vi "_Main_ByRuns_DAC2022_V1.0.1.vi"() -> ()   [LabVIEW 2017]
uses:
  <vilib>/Instr/_visa.llb/VISA Configure Serial Port (Instr).vi
panel:
  out "Field, kV/cm":dbl
  out "Current, mA":dbl
  out "Voltage, V":dbl
  in  "COM DAC":refnum<visa-resource-name>
  in  "WaveForm":i32(listbox)
  in  "Auto\nturn OFF":bool
  in  "Content":i32(listbox)
  out "LastTrigTimer, s":dbl
  in  "Graph every, cycle":dbl=10.0 min=1.0 max=100.0
  in  "SendPeriod, ms":dbl=100.0 min=10.0 max=10000.0
  out "RunsNeed":i32
  out "Time LOG":cluster{dbl[], dbl[]}(graph)
  out "TrigTimer, s":dbl
  out "Bytes at Port":u32
  out "RecTry":i32
  out "OutVoltage, V":dbl
  in  "Exposition, s":dbl=3.0
  out "Channel 2, V":dbl format="%#_5g"
  out "Channel 1, V":dbl format="%#_5g"
  in  "Stop Button":bool
  in  "Start Button":bool
  in  "Sample H, um":dbl=32.0
  out "VoltageArray, V":dbl[](array[numeric])
  out "Shutter Red":bool
  out "Shutter Green":bool
  in  "Frames In Run":u32=180
  out "Global Frame Done":u32
  out "Now is Run #":u32
  out "Frame In Run Done":u32
  in  "Step, kV/cm":dbl=1.0 min=0.01 max=1000.0
  in  "Amplitude, kV/cm":dbl=10.0 min=10.0 max=1500.0
  in  "LOG file":path
  in  "COM ADC":refnum<visa-resource-name>
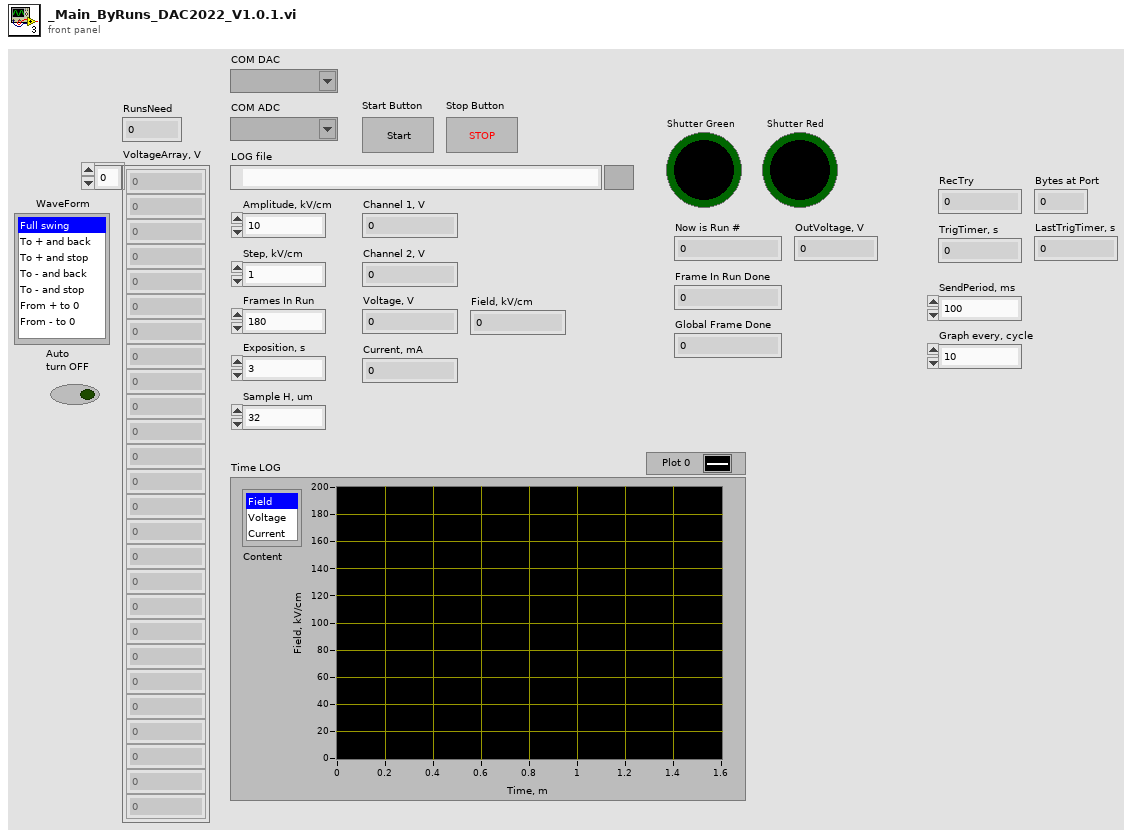
[diagram p1: front panel]
types:
  T1 = cluster{i32, i32, u32, "TrigState":bool, "TrigTimer, s":dbl, "CurrentError":bool}
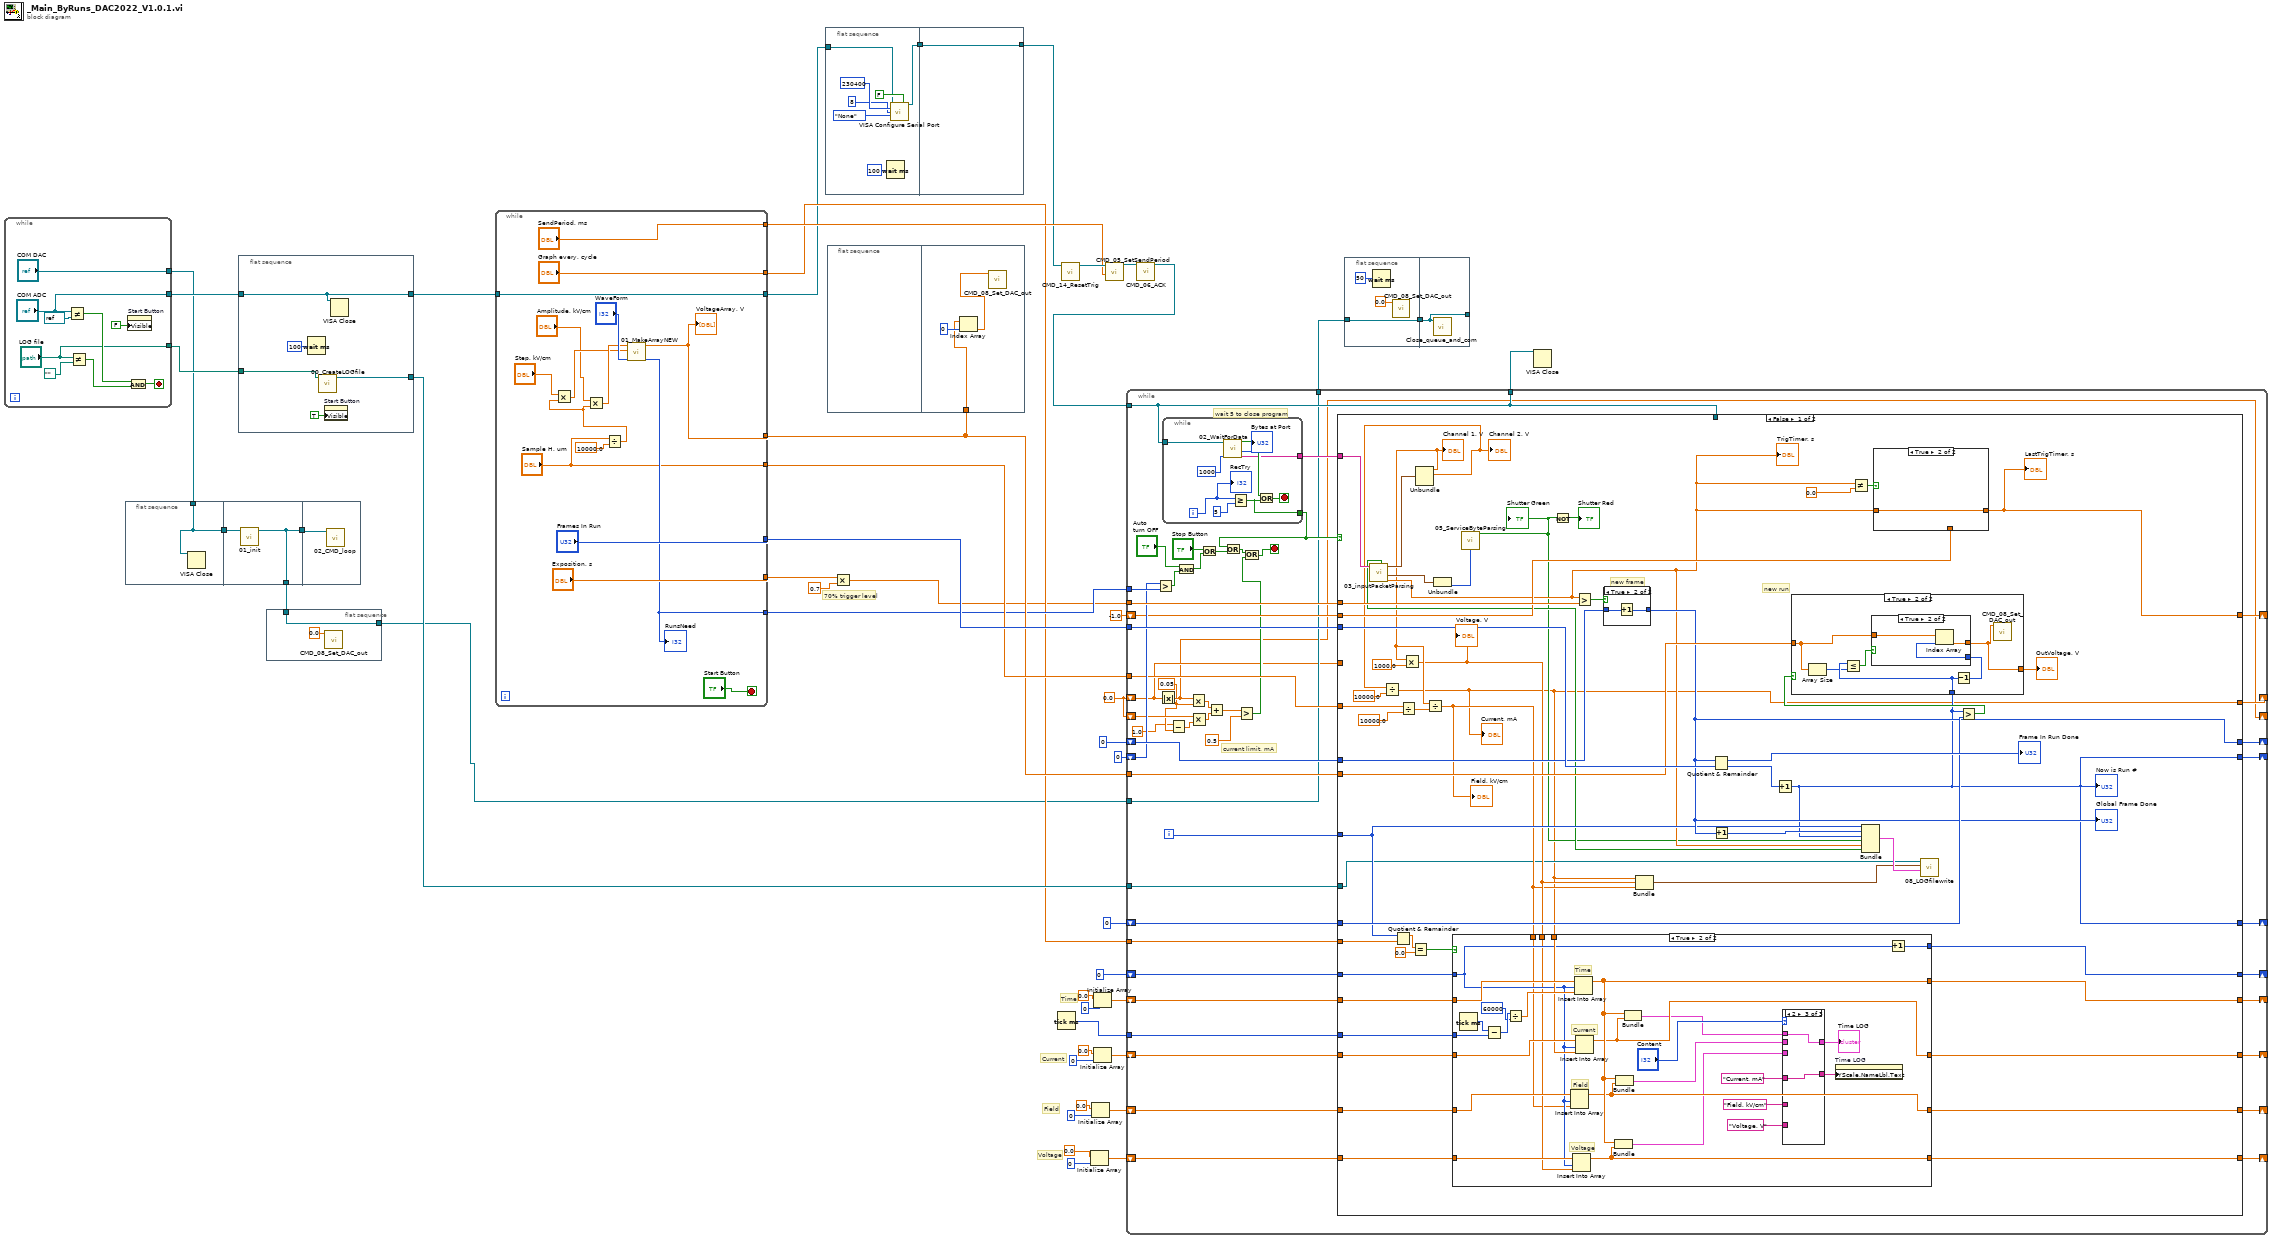
[diagram p0: block diagram]
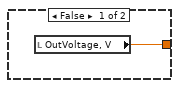
[diagram p6: hidden frame]
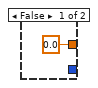
[diagram p7: hidden frame]
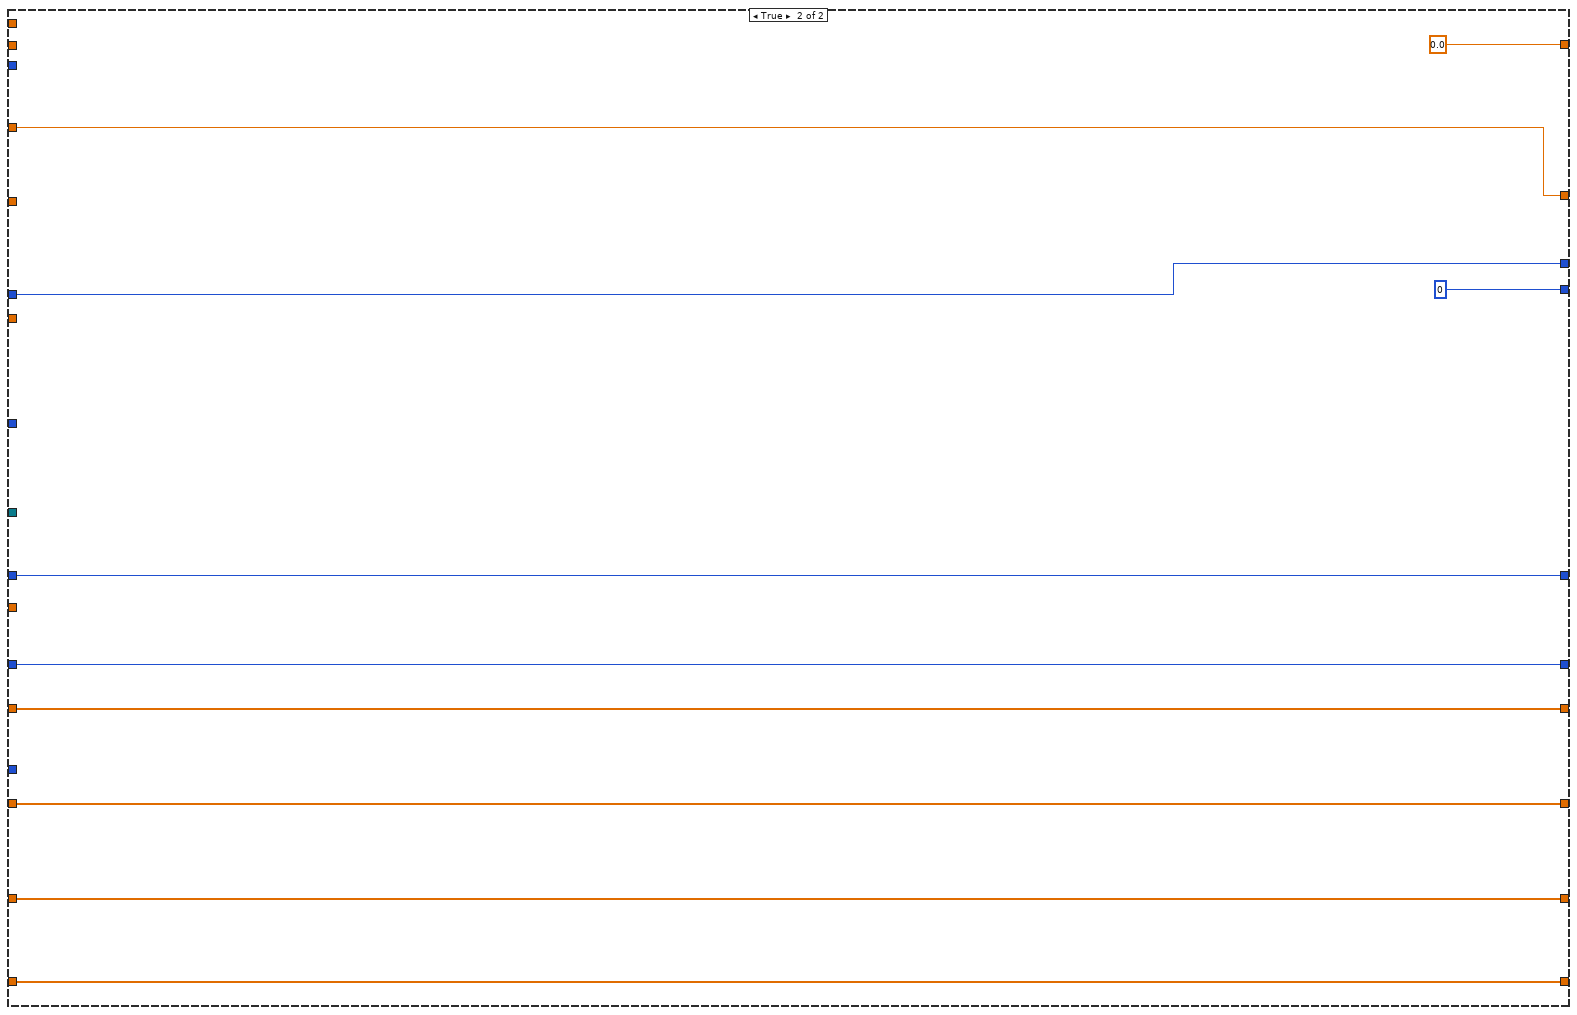
[diagram p9: hidden frame]
diagram:
  w1 = 0.0
  # "70% trigger level"
  # "Voltage"
  # "Field"
  # "Time"
  # "Current"
  n1 = while {
    tunnel: ["COM ADC"] -> w15
    tunnel: ["LOG file"] -> w14
    tunnel: ["COM DAC"] -> w6
    stop <- w53 stop-if-true
    n2 = Not Equal?(x="COM ADC", y=refnum<visa-resource-name> refnum ("COM port")) -> (x != y?=w50:bool)
    n3 = Not Equal?(x="LOG file", y=path "" ("LOG file")) -> (x != y?=w51:bool)
    n4 = property on="Start Button" class="Bool"("Visible"=FALSE) -> ()  [unwired: 2 in, 2 out]
    n5 = And(x=w50, y=w51) -> (x .and. y?=w53:bool)
  }
  n6 = flat-sequence {
    tunnel: [w56] -> w8
    tunnel: w6 -> [w56]
    tunnel: w8 -> [w58]
    tunnel: [w57] -> w5
    tunnel: [w57] -> w7
    tunnel: w7 -> [w59]
    frame #0 {
      n7 = VISA Close(VISA resource name=w56) -> ()  [unwired: 1 in, 1 out]
    }
    frame #1 {
      n8 = call "01_init.vi"("COM port"=w58) -> ("VISA resource name out"=w57:refnum<visa-resource-name>)  [unwired: 8 in, 2 out]
    }
    frame #2 {
      n9 = call "02_CMD_loop.vi"("VISA resource name"=w59) -> ()  [unwired: 11 in]
    }
  }
  n10 = flat-sequence {
    tunnel: [w64] -> w44
    tunnel: w15 -> [w60]
    tunnel: w14 -> [w61]
    tunnel: [w60] -> w13
    frame #0 {
      n11 = Wait (ms)(milliseconds to wait=u32 100) -> ()  [unwired: 1 out]
      n12 = call "00_CreateLOGfile.vi"("LOG file"=w61) -> ("refnum out"=w64:refnum<file>)  [unwired: 10 in]
      n13 = property on="Start Button" class="Bool"("Visible"=TRUE) -> ()  [unwired: 2 in, 2 out]
      n14 = VISA Close(VISA resource name=w60) -> ()  [unwired: 1 in, 1 out]
    }
  }
  n15 = flat-sequence {
    tunnel: w5 -> [w65]
    tunnel: [w65] -> w2
    frame #0 {
      n16 = call "CMD_08_Set_DAC_out.vi"("DAC voltage, V"=0.0) -> ()  [unwired: 11 in]
    }
  }
  n17 = while {
    tunnel: w13 -> [w76]
    tunnel: [w76] -> w11
    tunnel: [w75] -> w38
    tunnel: ["Sample H, um"] -> w45
    tunnel: ["Frames In Run"] -> w46
    tunnel: ["Exposition, s"] -> w24
    tunnel: [w74] -> w29
    tunnel: ["SendPeriod, ms"] -> w27
    tunnel: ["Graph every, cycle"] -> w26
    stop <- "Start Button" stop-if-true
    n18 = Divide(x="Sample H, um", y=10000.0) -> (x/y=w68:dbl)
    n19 = Multiply(x="Step, kV/cm", y=w68) -> (x*y=w70:dbl)
    n20 = Multiply(x="Amplitude, kV/cm", y=w68) -> (x*y=w71:dbl)
    n21 = call "01_MakeArrayNEW.vi"("Amp"=w71, "Step"=w70, "WaveForm"="WaveForm") -> ("Array"=w75:dbl[], "ArraySize"=w74:i32)  [unwired: 6 in]
    "VoltageArray, V" <- w75
    "RunsNeed" <- w74
  }
  n22 = flat-sequence {
    tunnel: w11 -> [w85]
    tunnel: [w84] -> w12
    tunnel: w12 -> [w90]
    tunnel: [w90] -> w10
    frame #0 {
      n23 = Wait (ms)(milliseconds to wait=u32 100) -> ()  [unwired: 1 out]
      n24 = call-poly "VISA Configure Serial Port"("VISA resource name"=w85, "Enable Termination\nChar (T)"=FALSE ("Enable Termination\nChar (T)"), "baud rate (9600)"=u32 230400, "data bits (8)"=u16 8, "parity (0:none)"=enum16{"None", "Odd", "Even", "Mark", "Space"}."None") -> ("VISA resource name out"=w84:refnum<visa-resource-name>)  [unwired: 9 in, 1 out]
    }
    frame #1 {
    }
  }
  n25 = flat-sequence {
    tunnel: w38 -> [w92]
    frame #0 {
    }
    frame #1 {
      n26 = Index Array(array=w92, index=0) -> (element=w91:dbl)
      n27 = call "CMD_08_Set_DAC_out.vi"("DAC voltage, V"=w91) -> ()  [unwired: 11 in]
    }
  }
  n28 = Multiply(x=w24, y=0.7) -> (x*y=w25:dbl)
  n29 = Tick Count (ms)() -> (millisecond timer value=w33:u32)
  n30 = call "CMD_14_ResetTrig.vi"("VISA resource name"=w10) -> ("VISA resource name out"=w41:refnum<visa-resource-name>)  [unwired: 10 in]
  n31 = Initialize Array(0.0 ("element"), 0 ("dimension size")) -> (w16:dbl[])
  n32 = Initialize Array(0.0 ("element"), 0 ("dimension size")) -> (w17:dbl[])
  n33 = Initialize Array(0.0 ("element"), 0 ("dimension size")) -> (w30:dbl[])
  n34 = Initialize Array(0.0 ("element"), 0 ("dimension size")) -> (w34:dbl[])
  n35 = call "CMD_05_SetSendPeriod.vi"("Period, ms"=w27, "VISA resource name"=w41) -> ("VISA resource name out"=w40:refnum<visa-resource-name>)  [unwired: 9 in]
  n36 = call "CMD_06_ACK.vi"("VISA resource name"=w40) -> ("VISA resource name out"=w39:refnum<visa-resource-name>)  [unwired: 10 in]
  n37 = while {
    tunnel: w39 -> [w110]
    tunnel: w38 -> [w133]
    tunnel: w46 -> [w139]
    tunnel: w25 -> [w141]
    tunnel: w45 -> [w111]
    tunnel: w44 -> [w140]
    shift-right: [w136] -> _
    shift-left: 0 -> [w138]
    shift-right: [w135] -> _
    shift-left: u32 0 -> [w134]
    shift-right: [w131] -> _
    shift-left: 0 -> [w132]
    tunnel: w33 -> [w129]
    shift-right: [w127] -> _
    shift-left: w34 -> [w130]
    shift-right: [w126] -> _
    shift-left: w30 -> [w128]
    tunnel: w29 -> [w122]
    shift-right: [w124] -> _
    shift-left: u32 0 -> [w121]
    tunnel: w26 -> [w118]
    shift-right: [w117] -> _
    shift-left: -1.0 ("TrigTimer, s") -> [w116]
    shift-right: [w113] -> _
    shift-left: w17 -> [w115]
    shift-right: [w112] -> _
    shift-left: w16 -> [w114]
    tunnel: [w109] -> w3
    tunnel: [w110] -> w9
    tunnel: w2 -> [w109]
    shift-right: [w108] -> _
    shift-left: w1 -> [w103]
    shift-right: [w102] -> _
    shift-left: w1 -> [w101]
    i -> [w137]
    stop <- w106 stop-if-true
    w99 = 0.05
    # "current limit, mA"
    # "wait 5 to close program"
    n38 = Greater?(x=w121, y=w122) -> (0:w119:bool)
    n39 = Absolute Value(x=w103) -> (abs(x)=w102:dbl)
    n40 = while {
      tunnel: w110 -> [w262]
      tunnel: [w265] -> w143
      tunnel: [w266] -> w142
      i -> [w264]
      stop <- w268 stop-if-true
      n41 = call "02_WaitForData.vi"("WaitTimeoutMS"=u32 1000, "VISA"=w262) -> ("Buffer"=w266:string, "Bytes at Port"=→"Bytes at Port":u32, "Data Recived"=w267:bool)  [unwired: 7 in]
      n42 = Greater Or Equal?(x=w264, y=5) -> (x >= y?=w265:bool)
      n43 = Or(x=w267, y=w265) -> (x .or. y?=w268:bool)
      "RecTry" <- w264
    }
    n44 = Subtract(x=1.0, y=w99) -> (x-y=w100:dbl)
    n45 = And(x="Auto\nturn OFF", y=w119) -> (x .and. y?=w120:bool)
    n46 = Multiply(x=w102, y=w99) -> (x*y=w96:dbl)
    n47 = Multiply(x=w101, y=w100) -> (x*y=w97:dbl)
    n48 = Or(x="Stop Button", y=w120) -> (x .or. y?=w125:bool)
    n49 = Add(x=w96, y=w97) -> (x+y=w95:dbl)
    n50 = Or(x=w143, y=w125) -> (x .or. y?=w105:bool)
    n51 = Greater?(x=w95, y=0.5) -> (0:w104:bool)
    n52 = Or(x=w105, y=w104) -> (x .or. y?=w106:bool)
    n53 = case shown="False" w143 {
      tunnel: w142 -> [w197 _]
      tunnel: w141 -> [w193 _]
      tunnel: w140 -> [w145 _]
      tunnel: w139 -> [w194 _]
      tunnel: w138 -> [w191 w261]
      tunnel: w137 -> [w178 _]
      tunnel: [w183 w261] -> w136
      tunnel: [w169 w260] -> w135
      tunnel: w134 -> [w186 w260]
      tunnel: w133 -> [w187 _]
      tunnel: w110 -> [_ _]
      tunnel: w132 -> [w176 w259]
      tunnel: [w175 w259] -> w131
      tunnel: w130 -> [w174 w258]
      tunnel: w129 -> [w173 _]
      tunnel: w128 -> [w172 w257]
      tunnel: [w171 w258] -> w127
      tunnel: [w170 w257] -> w126
      tunnel: [w169 u32 0] -> w124
      tunnel: w118 -> [w168 _]
      tunnel: [w165 0.0 ("TrigTimer, s")] -> w117
      tunnel: w116 -> [w164 _]
      tunnel: w115 -> [w160 w254]
      tunnel: w114 -> [w159 w253]
      tunnel: [w158 w254] -> w113
      tunnel: [w157 w253] -> w112
      tunnel: w111 -> [w151 _]
      tunnel: [w144 w252] -> w108
      tunnel: w103 -> [_ w252]
      frame False {
        # "new run"
        # "new frame"
        n54 = call "03_inputPacketParsing.vi"("string"=w197) -> ("TrigTimer, s"=w163:dbl, "Service state"=w182:cluster{u8, u8}, "Voltage"=w195:cluster{dbl, dbl, dbl, dbl}, "CurrentError"=w162:bool)  [unwired: 6 in, 1 out]
        "TrigTimer, s" <- w163
        n55 = Quotient & Remainder(x=w178, y=w168) -> (x-y*floor(x/y)=w180:dbl)  [unwired: 1 out]
        n56 = Divide(x=w151, y=10000.0) -> (x/y=w152:dbl)
        n57 = Equal?(x=w180, y=0.0) -> (x = y?=w177:bool)
        n58 = Unbundle(w195) -> (w153:dbl, w155:dbl)  [unwired: 2 out]
        "Channel 1, V" <- w153
        "Channel 2, V" <- w155
        n59 = Divide(x=w155, y=10000.0) -> (x/y=w144:dbl)
        "Current, mA" <- w144
        n60 = Multiply(x=w153, y=1000.0) -> (x*y=w148:dbl)
        "Voltage, V" <- w148
        n61 = Divide(x=w153, y=w152) -> (x/y=w147:dbl)
        "Field, kV/cm" <- w147
        n62 = Unbundle(w182) -> (w181:u8)  [unwired: 1 out]
        n63 = case shown="True" w177 {
          tunnel: w176 -> [w204 w220]
          tunnel: [w204 w227] -> w175
          tunnel: w174 -> [w202 w225]
          tunnel: w173 -> [_ w230]
          tunnel: w172 -> [w203 w224]
          tunnel: [w203 w216] -> w170
          tunnel: [w202 w219] -> w171
          tunnel: w144 -> [_ w223]
          tunnel: w160 -> [w201 w222]
          tunnel: w159 -> [w200 w221]
          tunnel: [w201 w217] -> w158
          tunnel: [w200 w218] -> w157
          tunnel: w148 -> [_ w206]
          tunnel: w147 -> [_ w205]
          frame False {
          }
          frame True {
            # "Time"
            # "Voltage"
            # "Field"
            # "Current"
            n64 = Tick Count (ms)() -> (millisecond timer value=w231:u32)
            n65 = Subtract(x=w231, y=w230) -> (x-y=w229:u32)
            n66 = Divide(x=w229, y=u32 60000) -> (x/y=w226:dbl)
            n67 = Insert Into Array(array=w222, index=w220, new element=w205) -> (w217:dbl[])
            n68 = Insert Into Array(array=w221, index=w220, new element=w206) -> (w218:dbl[])
            n69 = Insert Into Array(array=w225, index=w220, new element=w226) -> (w219:dbl[])
            n70 = Insert Into Array(array=w224, index=w220, new element=w223) -> (w216:dbl[])
            n71 = Bundle(w219, w218) -> (w212:cluster{dbl[], dbl[]})  [unwired: 1 in]
            n72 = Bundle(w219, w217) -> (w213:cluster{dbl[], dbl[]})  [unwired: 1 in]
            n73 = Bundle(w219, w216) -> (w214:cluster{dbl[], dbl[]})  [unwired: 1 in]
            n74 = case shown="2" "Content" {
              tunnel: w214 -> [_ _ w237]
              tunnel: w213 -> [w233 _ _]
              tunnel: w212 -> [_ w235 _]
              tunnel: [w233 w235 w237] -> w211
              tunnel: "Current, mA" ("Y Scale.Name Label.Text") -> [_ _ w236]
              tunnel: "Field, kV/cm" ("Y Scale.Name Label.Text") -> [w232 _ _]
              tunnel: "Voltage, V" ("Y Scale.Name Label.Text") -> [_ w234 _]
              tunnel: [w232 w234 w236] -> w207
              frame 0, Default {
              }
              frame 1 {
              }
              frame 2 {
              }
            }
            "Time LOG" <- w211
            n75 = property on="Time LOG" class="XYGraph (strict)"("YScale.NameLbl.Text"=w207) -> ()  [unwired: 2 in, 2 out]
            n76 = Increment(x=w220) -> (x+1=w227:i32)
          }
        }
        n77 = call "05_ServiceByteParsing.vi"("InputByte"=w181) -> ("TrigState"=w161:bool)  [unwired: 7 in, 3 out]
        "Shutter Green" <- w161
        n78 = Not(x=w161) -> (.not. x?=→"Shutter Red":bool)
        n79 = Greater?(x=w163, y=w193) -> (0:w192:bool)
        n80 = case shown="True" w192 {
          tunnel: w191 -> [w249 w251]
          tunnel: [w249 w250] -> w183
          frame False {
          }
          frame True {
            n81 = Increment(x=w251) -> (x+1=w250:i32)
          }
        }
        "Global Frame Done" <- w183
        n82 = Bundle(w144, w148, w147) -> (w146:cluster{dbl, dbl, dbl})  [unwired: 1 in]
        n83 = Quotient & Remainder(x=w183, y=w194) -> (x-y*floor(x/y)=→"Frame In Run Done":u32, floor(x/y)=w189:u32)
        n84 = Increment(x=w183) -> (x+1=w184:i32)
        n85 = Increment(x=w189) -> (x+1=w169:u32)
        "Now is Run #" <- w169
        n86 = Not Equal?(x=w163, y=0.0) -> (x != y?=w167:bool)
        n87 = Bundle(w178, w184, w169, "TrigState"=w161, "TrigTimer, s"=w163, "CurrentError"=w162) -> (w149:T1)  [unwired: 1 in]
        n88 = case shown="True" w167 {
          tunnel: [w198 w199] -> w165
          tunnel: w163 -> [_ w199]
          tunnel: w164 -> [w198 _]
          frame False {
          }
          frame True {
          }
        }
        "LastTrigTimer, s" <- w165
        n89 = call "08_LOGfilewrite.vi"("Counters"=w149, "output cluster"=w146, "refnum out"=w145) -> ()  [unwired: 9 in]
        n90 = Greater?(x=w169, y=w186) -> (0:w190:bool)
        n91 = case shown="True" w190 {
          tunnel: w187 -> [_ w240]
          tunnel: w169 -> [_ w243]
          tunnel: [w238 w239] -> w185
          frame False {
            n92 = local read "OutVoltage, V"() -> (w238:dbl)
          }
          frame True {
            n93 = Array Size(array=w240) -> (size(s)=w242:i32)
            n94 = Less Or Equal?(x=w243, y=w242) -> (x <= y?=w241:bool)
            n95 = Decrement(x=w243) -> (x-1=w244:u32)
            n96 = case shown="True" w241 {
              tunnel: w244 -> [_ w248]
              tunnel: w240 -> [_ w247]
              tunnel: [0.0 w246] -> w239
              frame False {
              }
              frame True {
                n97 = Index Array(array=w247, index=w248) -> (element=w246:dbl)
              }
            }
            n98 = call "CMD_08_Set_DAC_out.vi"("DAC voltage, V"=w239) -> ()  [unwired: 11 in]
          }
        }
        "OutVoltage, V" <- w185
      }
      frame True {
      }
    }
  }
  n99 = flat-sequence {
    tunnel: w3 -> [w272]
    tunnel: [w272] -> w4
    tunnel: [w274] -> _
    tunnel: w4 -> [w274]
    frame #0 {
      n100 = Wait (ms)(milliseconds to wait=u32 50) -> ()  [unwired: 1 out]
      n101 = call "CMD_08_Set_DAC_out.vi"("DAC voltage, V"=0.0) -> ()  [unwired: 11 in]
    }
    frame #1 {
      n102 = call "Close_queue_and_com.vi"("VISA"=w274) -> ()  [unwired: 11 in]
    }
  }
  n103 = VISA Close(VISA resource name=w9) -> ()  [unwired: 1 in, 1 out]
